vi "ResonanceCompensation.vi"(10 "Waveform Shape Fast Out":dbl[](array[numeric])) -> (1 "CorrectedWaveform":dbl[](graph), 2 "Outputs":waveform(dbl)[](graph), 3 "outWave":dbl[](graph))   [LabVIEW 2016]
uses:
  controls/Enum.ctl
  <vilib>/addons/Control Design/_Time Response Analysis/Time Response.llb/Time Response subVI/cd_Linear Simulation (Zero-Pole-Gain with Waveforms).vi
  <vilib>/addons/Control Design/_Time Response Analysis/NI_CD_Time Response.lvlib
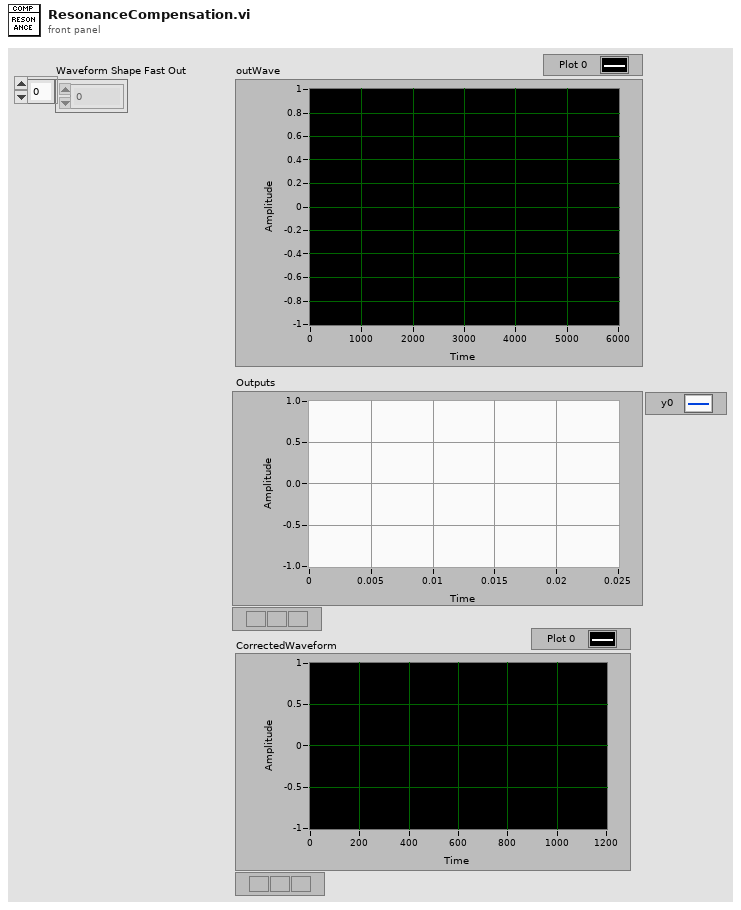
[diagram p1: front panel]
types:
  T1 = typedef "Enum.ctl" = enum16{"Init", "Read", "Write"}
  T2 = cluster{"outputRate":u16, "fastDecFactor":u16, "outWaveSizeFast":u16, "pplUpsampling":u16, "numLines":u16, "se.p.fastInvDec":fxp<+,22,0>, "se.p.slowUpStep":fxp<+,28,0>, "se.p.outWaveSizeSlow":u16, "blankingMax":u32, "se.p.fastBlanking":cluster{"startFwd":u32, "endFwd":u32, "startBwd":u32, "endBwd":u32, "disableBlanking":bool, "useCoarseCounter":bool}}
  T3 = cluster{"scanEngineHz":u32, "feedbackHz":u32, "sicmHz":u32, "rampHz":u32}
  T4 = typedef "NI_LinSys_Model Typedefs.lvlib/CD Zero-Pole-Gain Model (MIMO).ctl" = cluster{"properties":T5, "zero-pole-gain(s)":T6[][]}
  T5 = typedef "NI_LinSys_Model Typedefs.lvlib/CD General Elements.ctl" = cluster{"Model name":string, "Input names":string[], "Output names":string[], "Input Delays":dbl[], "Output Delays":dbl[], "Sampling Time":dbl, "Notes":string}
  T6 = typedef "NI_LinSys_Model Typedefs.lvlib/CD Zero-Pole-Gain Model (SISO).ctl" = cluster{"Gain":dbl, "Zeros":cdb[], "Poles":cdb[], "delay":dbl}
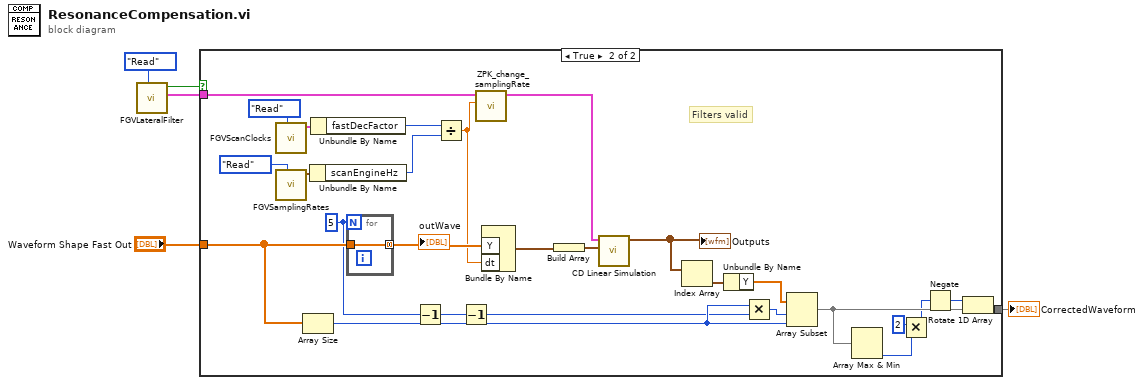
[diagram p0: block diagram]
diagram:
  n1 = call "FGVLateralFilter.vi"("Enum"=Enum."Read") -> ("ZPK input cluster 2"=w4:cluster{dbl, cdb[][], cdb[][], dbl}, "Filter valid output"=w1:bool)  [unwired: 6 in, 1 out]
  n2 = case shown="True" w1 {
    tunnel: w4 -> [_ w21]
    tunnel: "Waveform Shape Fast Out" -> [w6 w18]
    tunnel: [w6 w11] -> w2
    frame False {
    }
    frame True {
      w15 = 5
      # "Filters valid"
      n3 = call "FGVScanClocks.vi"("Enum"=Enum."Read") -> ("scanClocksOutput"=w32:T2)  [unwired: 7 in, 1 out]
      n4 = call "FGVSamplingRates.vi"("Enum"=Enum."Read") -> ("samplingRatesOut"=w33:T3)  [unwired: 9 in, 1 out]
      n5 = Array Size(array=w18) -> (size(s)=w16:i32)
      n6 = Unbundle By Name(w33) -> ("scanEngineHz"=w31:u32)
      n7 = Unbundle By Name(w32) -> ("fastDecFactor"=w30:u16)
      n8 = for {
        N: w15 -> [_]
        tunnel: [w34] -> w27 mode=concatenating
        tunnel: w18 -> [w34]
      }
      "outWave" <- w27
      n9 = Decrement(x=w15) -> (x-1=w14:i32)
      n10 = Divide(x=w30, y=w31) -> (x/y=w20:dbl)
      n11 = Decrement(x=w14) -> (x-1=w13:i32)
      n12 = call "ZPK_change_samplingRate.vi"("newSamplingTime"=w20, "ZPK input cluster in"=w21) -> ("Zero-Pole-Gain Model"=w19:T4)  [unwired: 9 in]
      n13 = Bundle By Name("Y"=w27, "dt"=w20) -> (w26:waveform(dbl))  [unwired: 1 in]
      n14 = Build Array(w26) -> (w25:waveform(dbl)[])
      n15 = call-poly <vilib>:"CD Linear Simulation.vi"("Inputs"=w25, "Zero-Pole-Gain Model"=w19) -> ("Outputs"=w24:waveform(dbl)[])  [unwired: 7 in, 2 out]
      "Outputs" <- w24
      n16 = Index Array(array=w24) -> (element=w23:waveform(dbl))  [unwired: 1 in]
      n17 = Unbundle By Name(w23) -> ("Y"=w22:dbl[])
      n18 = Multiply(x=w16, y=w13) -> (x*y=w17:i32)
      n19 = Array Subset(array=w22, index=w17, length=w16) -> (w12:dbl[])
      n20 = Array Max & Min(array=w12) -> (min index (indices)=w10:i32)  [unwired: 3 out]
      n21 = Multiply(x=2, y=w10) -> (x*y=w8:i32)
      n22 = Negate(x=w8) -> (-x=w9:i32)
      n23 = Rotate 1D Array(1:w12, 2:w9) -> (0:w11:dbl[])
    }
  }
  "CorrectedWaveform" <- w2
